vi "createNewLog.vi"(8 "error in (no error)":errorcluster, 11 "Model in":refnum<class "Model.lvclass">) -> (0 "error out":errorcluster, 3 "Model out":refnum<class "Model.lvclass">)   [LabVIEW 2013, in "Model.lvclass"]
uses:
  Model.lvclass
  Model.lvclass/Model.ctl
  ApplicationElements/Log/TestDataLog/TestDataLog.lvclass
  UserEvents/UserEvents.lvclass/UserEvents.ctl
  ApplicationElements/Log/StiffnessLog/StiffnessLog.lvclass
  <userlib>/Common/Log/Log/Log.lvclass/Log.ctl
  <userlib>/Common/Log/Log/Log.lvclass
  UserEvents/UserEvents.lvclass
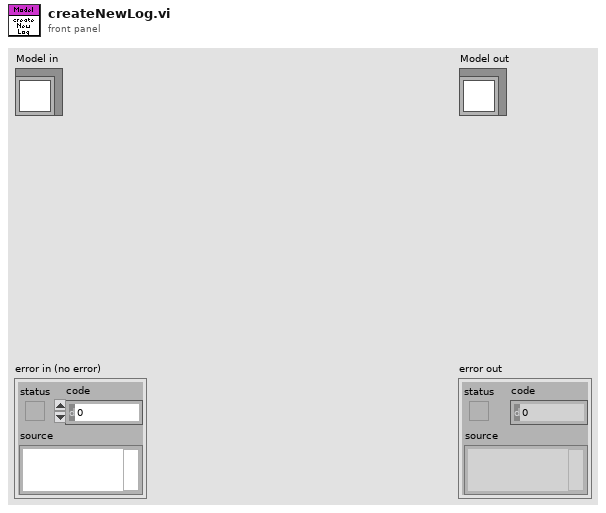
[diagram p1: front panel]
types:
  T1 = typedef "M2AADTTypedefs.lvlib/PubDataEvents.ctl" = cluster{"State":refnum<user-event>, "ErrorCode":refnum<user-event>, "OutputData":refnum<user-event>, "InputData":refnum<user-event>, "ControllerData":refnum<user-event>, "TestStatus":refnum<user-event>, "LogPath":refnum<user-event>, "StiffnessData":refnum<user-event>}
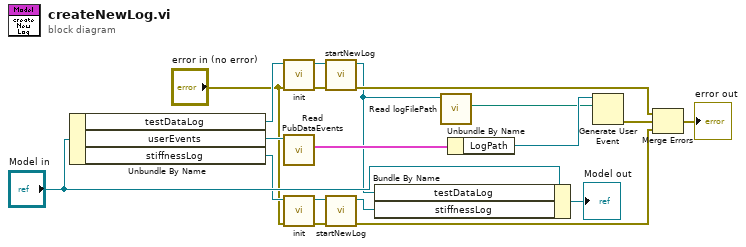
[diagram p0: block diagram]
diagram:
  n1 = Unbundle By Name("Model in") -> ("testDataLog"=w9:refnum<class "TestDataLog.lvclass">, "userEvents"=w12:refnum<class "UserEvents.lvclass">, "stiffnessLog"=w6:refnum<class "StiffnessLog.lvclass">)
  n2 = call-dynamic "init.vi"("error in (no error)"="error in (no error)", "Logger in"=w9) -> ("error out"=w7:errorcluster, "Logger out"=w8:refnum<class "TestDataLog.lvclass">)  [unwired: 8 in]
  n3 = call "Read PubDataEvents.vi"("UserEvents in"=w12) -> ("PubDataEvents"=w14:T1)  [unwired: 9 in, 1 out]
  n4 = call-dynamic "init.vi"("error in (no error)"="error in (no error)", "Logger in"=w6) -> ("error out"=w3:errorcluster, "Logger out"=w5:refnum<class "StiffnessLog.lvclass">)  [unwired: 8 in]
  n5 = call <userlib>:"startNewLog.vi"("error in (no error)"=w7, "Logger in"=w8) -> ("error out"=w17:errorcluster, "Logger out"=w10:refnum<class "TestDataLog.lvclass">)  [unwired: 8 in]
  n6 = call <userlib>:"startNewLog.vi"("error in (no error)"=w3, "Logger in"=w5) -> ("error out"=w2:errorcluster, "Logger out"=w4:refnum<class "StiffnessLog.lvclass">)  [unwired: 8 in]
  n7 = Bundle By Name(cluster="Model in", "testDataLog"=w10, "stiffnessLog"=w4) -> (→"Model out":refnum<class "Model.lvclass">)
  n8 = call <userlib>:"Read logFilePath.vi"("Logger in"=w10) -> ("logFilePath"=w11:path)  [unwired: 9 in, 1 out]
  n9 = Unbundle By Name(w14) -> ("LogPath"=w13:refnum<user-event>)
  n10 = Generate User Event(user event=w13, event data cluster=w11) -> (error out=w16:errorcluster)  [unwired: 2 in, 1 out]
  n11 = Merge Errors(w17, w16, w2) -> (→"error out":errorcluster)
